vi "Configure Analog In.vi"(0 "ADALM2000 Handler":u32 caption="Instrument Handle Out", 5 "Samplerate (Hz)":T2, 7 "analog_trigger_source":T1, 9 "Trigger enable":bool, 11 "analog_delay":i64) -> (4 "ADALM2000 Handler 2":u32 caption="Instrument Handle Out")   [LabVIEW 2015]
uses:
  Controls/SampleRateControlAin.ctl
  Controls/AnalogTriggerSource.ctl
  libm2k_lv.dll
panel:
  # "TRIGGER SETTINGS"
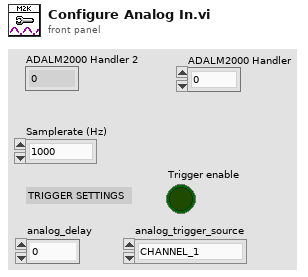
[diagram p1: front panel]
types:
  T1 = typedef "AnalogTriggerSource.ctl" = enum16{"CHANNEL_1", "CHANNEL_2", "CHANNEL_1_OR_CHANNEL_2", "CHANNEL_1_AND_CHANNEL_2", "CHANNEL_1_XOR_CHANNEL_2"}
  T2 = typedef "SampleRateControlAin.ctl" = enum16{"1000", "10000", "100000", "1000000", "10000000", "100000000"}
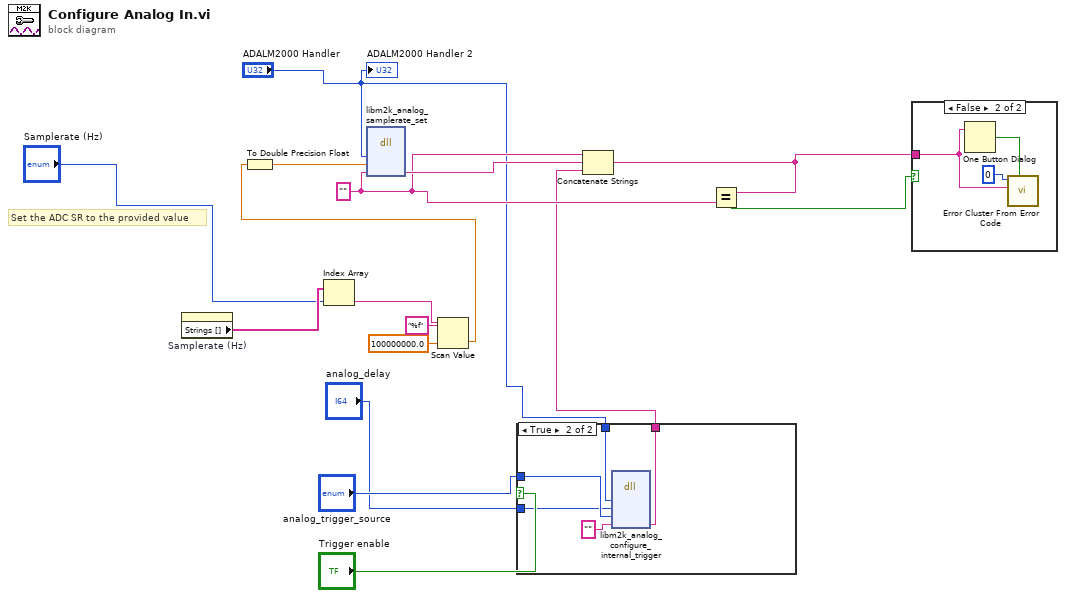
[diagram p0: block diagram]
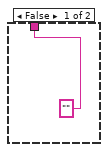
[diagram p2: hidden frame]
diagram:
  w14 = ""
  # "Set the ADC SR to the provided value"
  n1 = property on="Samplerate (Hz)" class="Enum (strict)"() -> ("Strings []"=w11:string[])  [unwired: 2 in, 2 out]
  n2 = Index Array(array=w11, index="Samplerate (Hz)") -> (element=w9:string)
  n3 = Scan Value(string=w9, format string="%f", default (0 dbl)=100000000.0) -> (value=w8:dbl)  [unwired: 1 out]
  n4 = To Double Precision Float(number=w8) -> (double precision float=w16:dbl)
  n5 = dll-call lib="libm2k_lv.*" fn="libm2k_analog_samplerate_set"("instance"="ADALM2000 Handler", "samplerate"=w16, "err"=w14) -> ("err"=w15:string)  [unwired: 6 in, 2 out]
  n6 = case shown="True" "Trigger enable" {
    tunnel: ["" ("err") w22] -> w4
    tunnel: "ADALM2000 Handler" -> [_ w21]
    tunnel: "analog_trigger_source" -> [_ w19]
    tunnel: "analog_delay" -> [_ w18]
    frame False {
    }
    frame True {
      n7 = dll-call lib="libm2k_lv.*" fn="libm2k_analog_configure_internal_trigger"("instance"=w21, "analog_delay"=w18, "analog_source"=w19, "err"="") -> ("err"=w22:string)  [unwired: 7 in, 2 out]
    }
  }
  n8 = Concatenate Strings(w14, w15, w4) -> (w12:string)
  n9 = Equal?(x=w12, y=w14) -> (x = y?=w13:bool)
  n10 = case shown="False" w13 {
    tunnel: w12 -> [_ w23]
    frame True {
    }
    frame False {
      n11 = One Button Dialog(message=w23) -> (true=w25:bool)  [unwired: 1 in]
      n12 = call <vilib>:"Error Cluster From Error Code.vi"("show call chain? (False)"=w25, "error message (\"\")"=w23, "error code (0)"=0) -> ()  [unwired: 6 in, 1 out]
    }
  }
  "ADALM2000 Handler 2" <- "ADALM2000 Handler"
